vi "OE1311&OE1351_Ethernet_Query Data.vi"(5 "Connection ID in":refnum<k5>, 7 "Timeout":u32=1000, 11 "Error in (no error)":errorcluster caption="error out（no error）") -> (3 "Buffer Count":u8, 4 "Connection ID out":refnum<k5>, 6 "Total Date Array":dbl[][](array[numeric]), 8 "Parameter Values":T2, 10 "Output String":string, 13 "Trig_Count":u8[](array[numeric]), 14 "PLL&Overload":T1, 15 "Error out":errorcluster caption="error out")   [LabVIEW 2011]
panel:
  out "Read Buffer":string
  in  "buffer":string
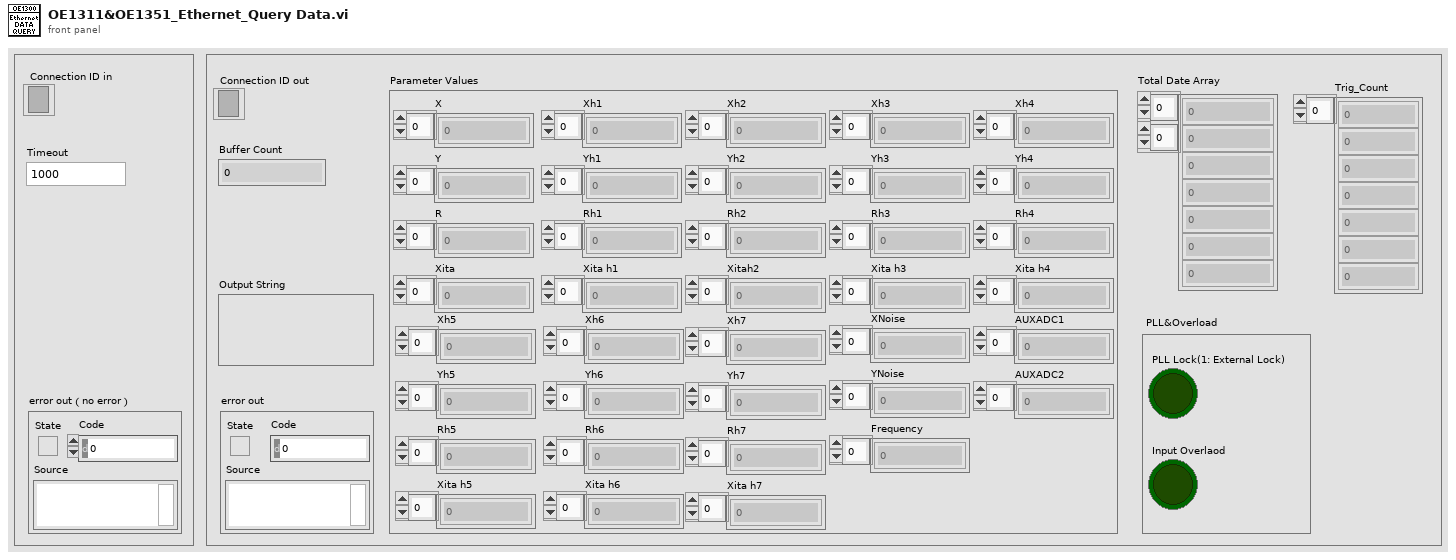
[diagram p1: front panel]
types:
  T1 = cluster{"PLL Lock(1: External Lock)":bool, "Input Overlaod":bool}
  T2 = cluster{"X":dbl[], "Y":dbl[], "R":dbl[], "Xita":dbl[], "XNoise":dbl[], "YNoise":dbl[], "Frequency":dbl[], "Xh1":dbl[], "Yh1":dbl[], "Rh1":dbl[], "Xita h1":dbl[], "Xh2":dbl[], "Yh2":dbl[], "Rh2":dbl[], "Xitah2":dbl[], "Xh3":dbl[], "Yh3":dbl[], "Rh3":dbl[], "Xita h3":dbl[], "Xh4":dbl[], "Yh4":dbl[], "Rh4":dbl[], "Xita h4":dbl[], "Xh5":dbl[], "Yh5":dbl[], "Rh5":dbl[], "Xita h5":dbl[], "Xh6":dbl[], "Yh6":dbl[], "Rh6":dbl[], "Xita h6":dbl[], "Xh7":dbl[], "Yh7":dbl[], "Rh7":dbl[], "Xita h7":dbl[], "AUXADC1":dbl[], "AUXADC2":dbl[]}
  T3 = enum16{"ISRC", "IGND", "ICPL", "ILIN", "PHAS", "FMOD", "RSLP", "FREQ", "SWPT", "SLLM", "SULM", "SSLL", "SSLG", "STLM", "SWRM", "IRNG", "SENS", "RMOD", "OFLT", "OFSL", "SYNC", "DMOD", "HARM", "DARB", "SWVT", "SLVL", "SVLL", "SVUL", "SVSL", "SVSG", "SVTM", "SVRM", "RALL", "SNAP", "OUTP", "OAUX", "COUT", "CAUX", "COFP", "CEXP", "FPOP", "OEXP", "*IDN", "*RST", "OVLD", "INOV", "GNOV", "*PLL", "SSET", "RSET", "AGAN", "APHS", "ARSV", "ASCL", "EQCD", "EQCS", "SPED", "SRAT", "SLEN", "SSLE", "STRG", "SPRM", "STRD", "PAUS", "REST", "SPTS", "TRCA", "TEMP", "RSTU", "IHNZ", "DEQU", "SADD", "ARNG", "CSPE", "ISRCD", "IGNDD", "ICPLD", "ILIND", "PHASD", "FMODD", "RSLPD", "FREQD", "SWPTD", "SLLMD", "SULMD", "SSLLD", "SSLGD", "STLMD", "SWRMD", "SENSD", "RMODD", "OFLTD", "OFSLD", "SYNCD", "HARMD", "EQCDD", "EQCSD", "SNAPD", "OUTPD", "SWVTD", "SLVLD", "SVLLD", "SVULD", "SVSLD", "SVSGD", "SVTMD", "SVRMD", "SVDCD", "ARSVD", "AGAND", "APHSD", "ASCLD", "FPOPD", "CAUXD", "OEXPD", "SPEDD", "SRATD", "SLEND", "SSLED", "STRGD", "SPRMD", "STRDD", "PAUSD", "RESTD", "SPTSD", "TRCAD", "*IDND", "*RSTD", "INOVD", "GNOVD", "*PLLD", "SSETD", "RSETD", "RALLD"}
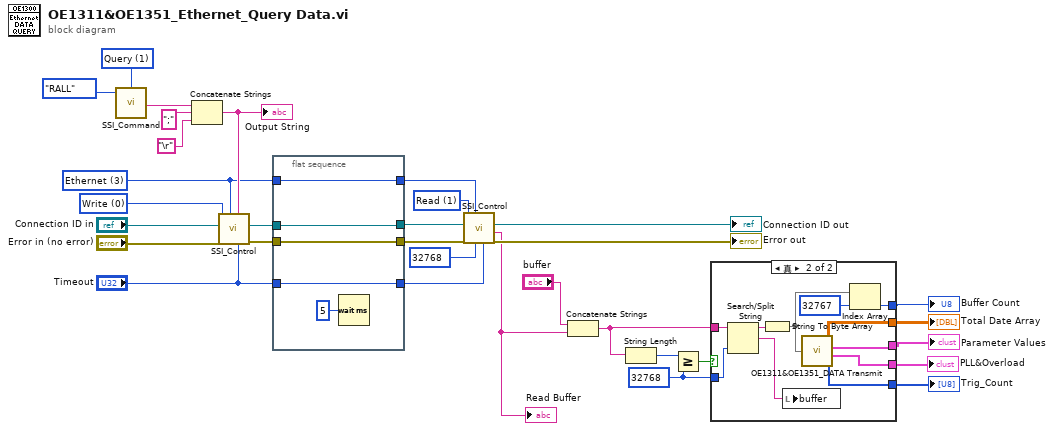
[diagram p0: block diagram]
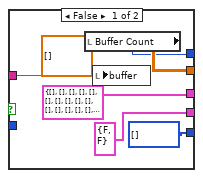
[diagram p2: hidden frame]
diagram:
  w1 = 32768 ("y")
  w12 = u16 3 items=["USB", "RS232", "GPIB", "Ethernet"] ("Remote Mode")
  w26 = u16 1 items=["Set", "Query"] ("Opera")
  w8 = u16 1 items=["Write", "Read"] ("Control")
  w30 = u16 0 items=["Write", "Read"] ("Control")
  n1 = call "SSI_Command.vi"("Opera"=w26, "Command Type"=T3."RALL") -> ("Output string"=w25:string)  [unwired: 2 in]
  n2 = Concatenate Strings(w25, ";" ("字符串"), "\r") -> (w29:string)
  "Output String" <- w29
  n3 = call "SSI_Control.vi"("Tineout"="Timeout", "Write Buffer"=w29, "Remote Mode"=w12, "Error in (no error)"="Error in (no error)", "Control"=w30, "Connection ID in"="Connection ID in") -> ("Error out"=w16:errorcluster, "Connection ID out"=w14:refnum<k5>)  [unwired: 2 in, 2 out]
  n4 = flat-sequence {
    tunnel: [w37] -> w10
    tunnel: "Timeout" -> [w37]
    tunnel: w16 -> [w36]
    tunnel: [w36] -> w15
    tunnel: [w35] -> w13
    tunnel: w14 -> [w35]
    tunnel: [w34] -> w11
    tunnel: w12 -> [w34]
    frame #0 {
      n5 = Wait (ms)(milliseconds to wait=u32 5 ("等待时间（毫秒）")) -> ()  [unwired: 1 out]
    }
  }
  n6 = call "SSI_Control.vi"("Tineout"=w10, "Number of bytes"=u32 32768, "Remote Mode"=w11, "Error in (no error)"=w15, "Control"=w8, "Connection ID in"=w13) -> ("Error out"=→"Error out":errorcluster, "Read Buffer"=w4:string, "Connection ID out"=→"Connection ID out":refnum<k5>)  [unwired: 2 in, 1 out]
  "Read Buffer" <- w4
  n7 = Concatenate Strings("buffer", w4) -> (w2:string)
  n8 = String Length(string=w2) -> (length=w3:i32)
  n9 = Greater Or Equal?(x=w3, y=w1) -> (x >= y?=w18:bool)
  n10 = case shown="真" w18 {
    tunnel: [T2 {"X"=[], "Y"=[], "R"=[], "Xita"=[], "XNoise"=[], "YNoise"=[], "Frequency"=[], "Xh1"=[], "Yh1"=[], "Rh1"=[], "Xita h1"=[], "Xh2"=[], "Yh2"=[], "Rh2"=[], "Xitah2"=[], "Xh3"=[], "Yh3"=[], "Rh3"=[], "Xita h3"=[], "Xh4"=[], "Yh4"=[], "Rh4"=[], "Xita h4"=[], "Xh5"=[], "Yh5"=[], "Rh5"=[], "Xita h5"=[], "Xh6"=[], "Yh6"=[], "Rh6"=[], "Xita h6"=[], "Xh7"=[], "Yh7"=[], "Rh7"=[], "Xita h7"=[], "AUXADC1"=[], "AUXADC2"=[]} ("Parameter Values") w51] -> w21
    tunnel: [dbl[][] [] ("Total Data Array") w52] -> w22
    tunnel: [w38 w53] -> w23
    tunnel: [u8[] [] ("Trig_Count") w50] -> w20
    tunnel: [T1 {"PLL Lock(1: External Lock)"=FALSE, "Input Overlaod"=FALSE} ("PLL&Overload") w49] -> w19
    tunnel: w2 -> [w39 w47]
    tunnel: w1 -> [_ w46]
    frame False {
      n11 = local read "Buffer Count"() -> (w38:u8)
      n12 = local write "buffer"(w39) -> ()
    }
    frame True {
      n13 = Search/Split String(string=w47, offset (0)=w46) -> (substring before match=w45:string, match + rest of string=w44:string)  [unwired: 1 in, 1 out]
      n14 = String To Byte Array(string=w45) -> (unsigned byte array=w48:u8[])
      n15 = local write "buffer"(w44) -> ()
      n16 = call "OE1311&OE1351_DATA Transmit.vi"("Input Data"=w48) -> ("Total Date Array"=w52:dbl[][], "Parameter Values"=w51:T2, "PLL&Overload"=w49:T1, "Trig_Count"=w50:u8[])
      n17 = Index Array(array=w48, index=32767 ("索引")) -> (element=w53:u8)
    }
  }
  "Parameter Values" <- w21
  "Total Date Array" <- w22
  "Buffer Count" <- w23
  "PLL&Overload" <- w19
  "Trig_Count" <- w20
